vi "myFreqPreview.vi"(4 "f_tick_min":u32, 5 "同步频率上限 f_tick_ref":u32=1 min=1 max=50, 6 "f_mes_max":u32, 7 "测量周期数 n":u32=2 min=1 max=10, 8 "freqs, measu, comps":i32[][](array[numeric]), 9 "index group":i32[][](array[numeric]), 10 "freqs groups":i32[][][](array[numeric])) -> (0 "最大同时使用内存(kS)":u64 caption="单频点最大使用内存(kS)", 1 "扫频点密度及其采样时长预览":T1(graph), 3 "group报告":string)   [LabVIEW 2024]
doc: "根据频率组，生成它的文本形式、xy图形式预览。"
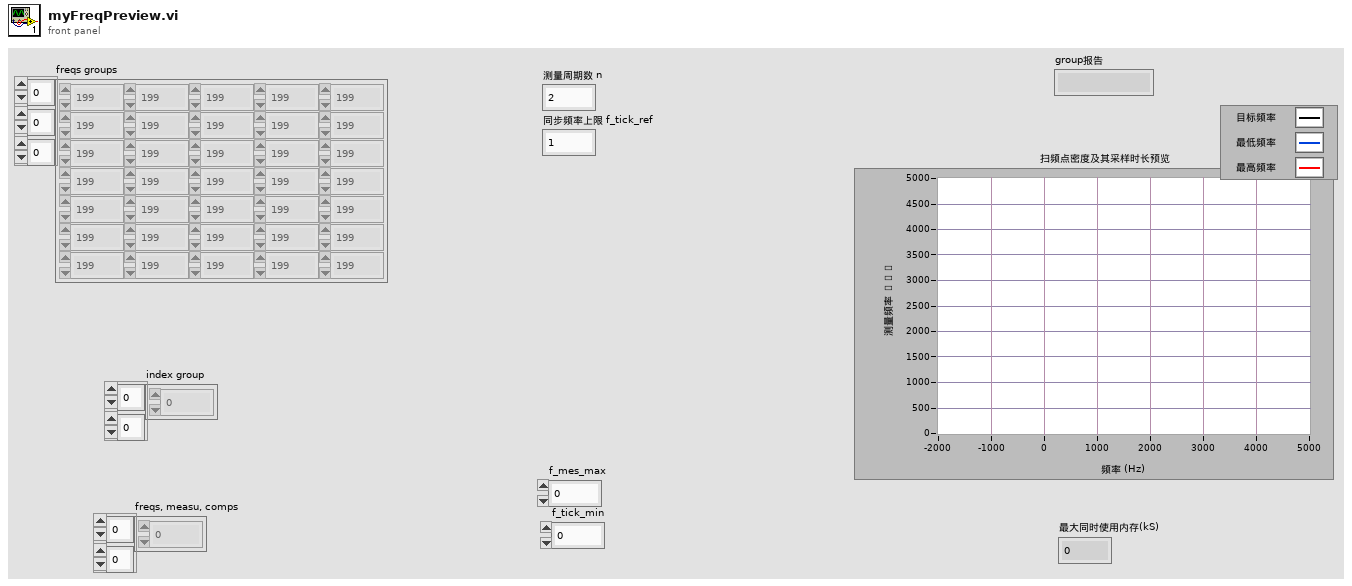
[diagram p1: front panel]
types:
  T1 = cluster{"freqs, measu, measu comp":i32[], dbl[]}[]
  T2 = cluster{"freqs, measu, comps":i32[], "freqs, measu, comps":i32[]}
  T3 = cluster{"freqs, measu, comps":i32[], "freqs, measu, comps":dbl[]}[]
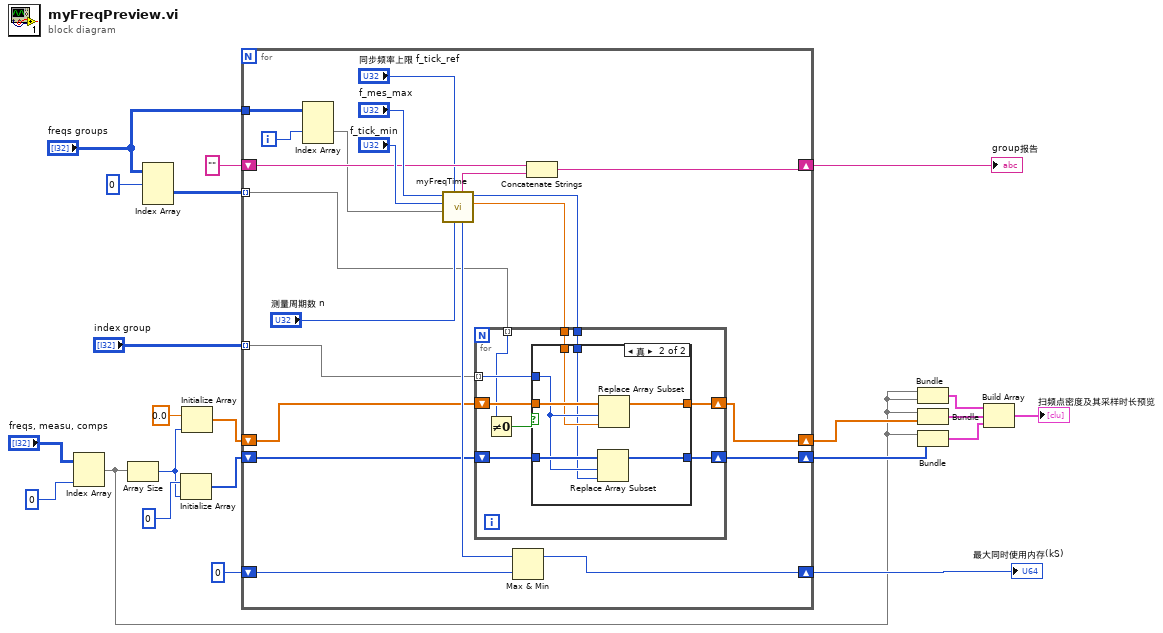
[diagram p0: block diagram]
diagram:
  n1 = Index Array(array="freqs, measu, comps", index (col)=0) -> (element=w6:i32[])  [unwired: 1 in]
  n2 = Array Size(array=w6) -> (size(s)=w9:i32)
  n3 = Index Array(array="freqs groups", index (dim 0)=0 ("索引 (页)")) -> (element=w2:i32[][])  [unwired: 2 in]
  n4 = Initialize Array(u32 0, w9) -> (w18:u32[])
  n5 = Initialize Array(0.0, w9) -> (w19:dbl[])
  n6 = for {
    tunnel: "index group" -> [w33] mode=indexing
    shift-right: [w39] -> w5
    shift-left: "" -> [w40]
    shift-right: [w35] -> w20
    shift-left: u32 0 -> [w36]
    shift-right: [w28] -> w8
    shift-left: w19 -> [w32]
    shift-right: [w27] -> w7
    shift-left: w18 -> [w31]
    tunnel: w2 -> [w26] mode=indexing
    tunnel: "freqs groups" -> [w25]
    i -> [w23]
    n7 = Index Array(array=w25, index (dim 1)=w23) -> (element=w24:i32[][])  [unwired: 2 in]
    n8 = call "myFreqTime.vi"("测量周期数 n"="测量周期数 n", "同步频率上限 f_tick_ref"="同步频率上限 f_tick_ref", "freqs rows"=w24, "f_tick_min"="f_tick_min", "f_mes_max"="f_mes_max") -> ("f_tick"=w30:dbl, "f_mes"=w29:i32, "mem_size"=w37:u32, "row报告"=w41:string)  [unwired: 1 in, 2 out]
    n9 = for {
      tunnel: w33 -> [w50] mode=indexing
      tunnel: w26 -> [w48] mode=indexing
      tunnel: w30 -> [w47]
      tunnel: w29 -> [w46]
      shift-right: [w45] -> w28
      shift-left: w32 -> [w52]
      shift-right: [w44] -> w27
      shift-left: w31 -> [w51]
      n10 = Not Equal To 0?(x=w48) -> (x != 0?=w49:bool)
      n11 = case shown="真" w49 {
        tunnel: w52 -> [w54 w61]
        tunnel: w51 -> [w53 w60]
        tunnel: w50 -> [_ w59]
        tunnel: w47 -> [_ w58]
        tunnel: w46 -> [_ w57]
        tunnel: [w54 w56] -> w45
        tunnel: [w53 w55] -> w44
        frame False {
        }
        frame True {
          n12 = Replace Array Subset(array=w60, new element=w57, index=w59) -> (w55:u32[])
          n13 = Replace Array Subset(array=w61, new element=w58, index=w59) -> (w56:dbl[])
        }
      }
    }
    n14 = Max & Min(x=w37, y=w36) -> (max(x,y)=w35:u32)  [unwired: 1 out]
    n15 = Concatenate Strings(w40, w41) -> (w39:string)
  }
  "最大同时使用内存(kS)" <- w20
  "group报告" <- w5
  n16 = Bundle("freqs, measu, comps"=w6, "freqs, measu, comps"=w6) -> (w14:T2)  [unwired: 1 in]
  n17 = Bundle("freqs, measu, comps"=w6, w8) -> (w13:cluster{"freqs, measu, comps":i32[], dbl[]})  [unwired: 1 in]
  n18 = Bundle("freqs, measu, comps"=w6, w7) -> (w12:cluster{"freqs, measu, comps":i32[], u32[]})  [unwired: 1 in]
  n19 = Build Array(w14, w13, w12) -> (→"扫频点密度及其采样时长预览":T3)
